vi "DataConcat.vi"() -> ()   [LabVIEW 2015]
panel:
  out "error out":errorcluster
  in  "Path":path=path "C:/Users/leser/Dropbox/Equipo9/Activity_6.vi"
  in  "Boolean":bool
  in  "initial string 2":string="Luis Esteban Serrano"
  in  "initial string":string="Name: "
  out "resulting string":string="Name: Luis Esteban Serrano\nC:\\Users\\leser\\Dropbox\\Equipo9\\Activity_6.vi\n0"
  in  "format string":string="%s\\n%s\\n%d"
  # "Concatenacion de Diferentes tipos de Datos"
  # "Serrano Bermúdez Luis Esteban\nFecha de Entrega 17/02/2019"
  # "Descripcion: Esta aplicacion une distintos tipos de datos en una sola cadena\nstring, donde serán mostrados dependiendo del indicador con el que sea \nespecificado."
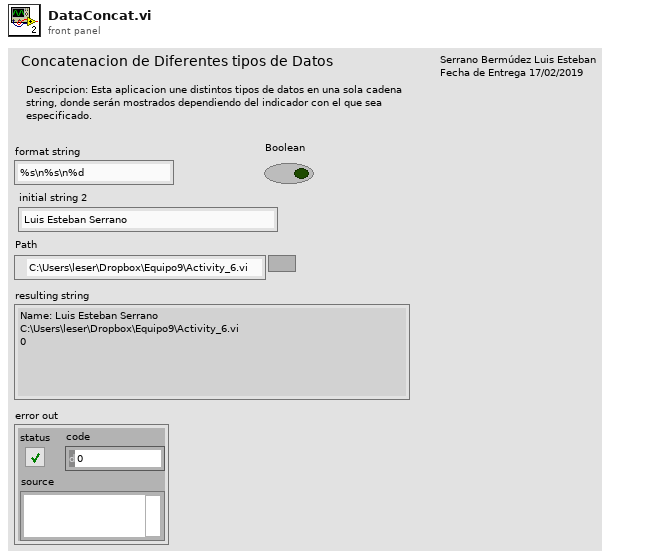
[diagram p1: front panel]
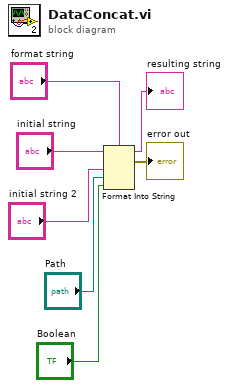
[diagram p0: block diagram]
diagram:
  n1 = Format Into String(format string="format string", initial string="initial string", "initial string 2", "Path", "Boolean") -> (resulting string=→"resulting string":string, error out=→"error out":errorcluster)  [unwired: 1 in]
